vi "MH_LibVersion_global.vi"() -> ()   [LabVIEW 2019]
panel:
  in  "Library Version":string="3.0"
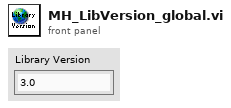
[diagram p1: front panel]
diagram:
